vi "PhotonPoseEstimator_New.vi"(6 "BaseNTName":string="/photonvision", 8 "RobotToCamera":T1={"TRANSLATION3D"={"X"=0.0, "Y"=0.0, "Z"=0.0}, "ROTATION3D"={"Q_quaternion"={"R"=1.0, "V"=[0.0, 0.0, 0.0]}}, "XF"=FALSE} {"TRANSLATION3D"."Z" format="%14.3f"; "TRANSLATION3D"."Y" format="%14.3f"; "TRANSLATION3D"."X" format="%14.3f"}, 9 "Camera":string, 10 "Strategy":T5, 11 "AprilTagFieldLayout":T6={"AprilTagMap"={}, "FieldLength"=0.0, "FieldWidth"=0.0, "OriginPosition "=enum."kBlueAllianceWallRightSide,", "OriginPose3d"={"Translation3d"={"X"=0.0, "Y"=0.0, "Z"=0.0}, "Rotation3d"={"Q_quaternion"={"R"=1.0, "V"=[0.0, 0.0, 0.0]}}}} {"OriginPose3d"."Translation3d"."Z" format="%14.3f"; "OriginPose3d"."Translation3d"."Y" format="%14.3f"; "OriginPose3d"."Translation3d"."X" format="%14.3f"}) -> (3 "PhotonPoseEstimator":T10)   [LabVIEW 2019, in "PhotonVisionLib.lvlib"]
doc: "Create a new Photon Pose Estimator data cluster.\n\nThe PhotonPoseEstimator functions filters or combines readings from all the AprilTags visible at a given timestamp on the field to produce a single robot in field pose, using the strategy set below. Example usage can be found under the LabVIEW Find Examples..\n\nInputs:\n -- AprilTagFieldLayout -- cluster -- A WPILib LabVIEW Math cluster defining the absolute positions of April Tags on a FIRST field. with respect to the FIRST field \n -- Strategy -- Enum -- The strategy it should use to determine the best pose. Current strategies include:\n LOWEST_AMBIGUITY -- Choose the Pose with the lowest ambiguity\n CLOSEST_TO_CAMERA_HEIGHT -- Choose the Pose which is closest to the camera height.\n CLOSEST_TO_REFERENCE_POSE -- Choose the Pose which is closest to a set Reference position.\n CLOSEST_TO_LAST_POSE -- Choose the Pose which is closest to the last pose calculated\n AVERAGE_BEST_TARGETS -- Weight average of acceptable targets based on ambiguity..\n -- CameraName -- String -- Name of the photon camera.\n -- RobotToCamera -- Transform3d -- Transform from the center of the robot to the camera mount positions\n\nOutputs:\n -- PhotonPoseEstimator -- cluster -- created data cluster."
uses:
  PhotonVisionLib.lvlib
  Ref/PhotonPoseEstimator_REF.ctl
  TypeDef/PhotonPoseEstimatorType.ctl
  <vilib>/Rock Robotics/WPI/ThirdParty/JAS_Junk/TrajLib/TypeDef/POSE3D.ctl
  <vilib>/Rock Robotics/WPI/ThirdParty/JAS_Junk/TrajLib/TypeDef/TRANSLATION3D.ctl
  <vilib>/Rock Robotics/WPI/ThirdParty/JAS_Junk/TrajLib/TypeDef/ROTATION3D.ctl
  <vilib>/Rock Robotics/WPI/ThirdParty/JAS_Junk/TrajLib/TypeDef/QUATERNION.ctl
  <vilib>/Rock Robotics/WPI/ThirdParty/JAS_Junk/TrajLib/TypeDef/AprilTagFieldLayout.ctl
  <vilib>/Rock Robotics/WPI/ThirdParty/JAS_Junk/TrajLib/TypeDef/AprilTag.ctl
  <vilib>/Rock Robotics/WPI/ThirdParty/JAS_Junk/TrajLib/Enum/AprilTagFieldLayoutOrignPosition_ENUM.ctl
  Enum/PhotonPoseStrategy_ENUM.ctl
  <vilib>/Rock Robotics/WPI/ThirdParty/JAS_Junk/TrajLib/TypeDef/TRANSFORM3D.ctl
  TypeDef/PhotonTargetModel.ctl
  PhotonTargetModel_New_RectPlanar.vi
  <vilib>/Rock Robotics/WPI/ThirdParty/JAS_Junk/TrajLib/Conv_Inches_Meters.vi
  <vilib>/Rock Robotics/WPI/ThirdParty/JAS_Junk/TrajLib/VI/Translation3d_Create.vi
  PhotonTargetModel_New.vi
  <vilib>/Rock Robotics/WPI/ThirdParty/JAS_Junk/TrajLib/Trajectory_Library.lvlib
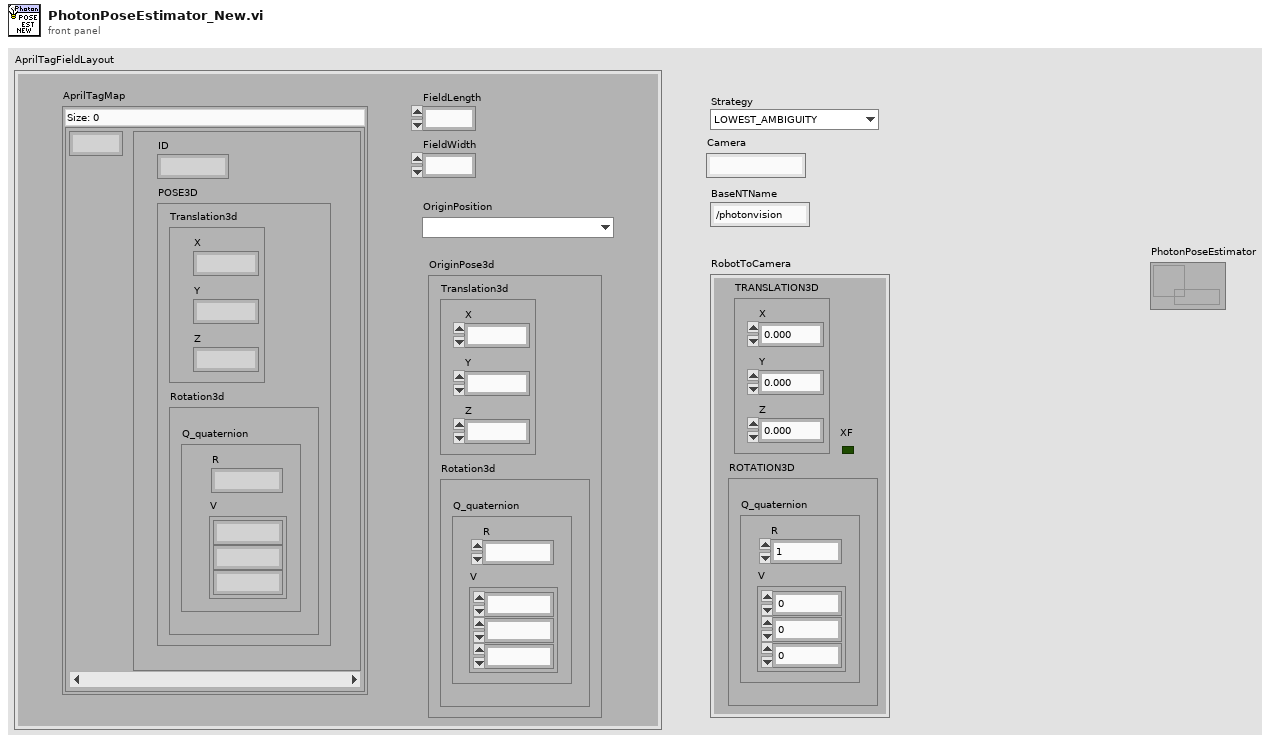
[diagram p1: front panel]
types:
  T1 = typedef "Trajectory_Library.lvlib/TRANSFORM3D.ctl" = cluster{"TRANSLATION3D":T2, "ROTATION3D":T3, "XF":bool}
  T2 = typedef "Trajectory_Library.lvlib/TRANSLATION3D.ctl" = cluster{"X":dbl, "Y":dbl, "Z":dbl}
  T3 = typedef "Trajectory_Library.lvlib/ROTATION3D.ctl" = cluster{"Q_quaternion":T4}
  T4 = typedef "Trajectory_Library.lvlib/QUATERNION.ctl" = cluster{"R":dbl, "V":dbl[]}
  T5 = typedef "PhotonVisionLib.lvlib/PhotonPoseStrategy_ENUM.ctl" = enum16{"LOWEST_AMBIGUITY", "CLOSEST_TO_CAMERA_HEIGHT", "CLOSEST_TO_REFERENCE_POSE", "CLOSEST_TO_LAST_POSE", "AVERAGE_BEST_TARGETS", "MULTI_TAG_PNP_ON_COPROCESSOR", "MULTI_TAG_PNP_ON_RIO"}
  T6 = typedef "Trajectory_Library.lvlib/AprilTagFieldLayout.ctl" = cluster{"AprilTagMap":map{i32, T7}, "FieldLength":dbl, "FieldWidth":dbl, "OriginPosition ":T9, "OriginPose3d":T8}
  T7 = typedef "Trajectory_Library.lvlib/AprilTag.ctl" = cluster{"ID":i32, "POSE3D":T8}
  T8 = typedef "Trajectory_Library.lvlib/POSE3D.ctl" = cluster{"Translation3d":T2, "Rotation3d":T3}
  T9 = typedef "Trajectory_Library.lvlib/AprilTagFieldLayoutOrignPosition_ENUM.ctl" = enum16{"kBlueAllianceWallRightSide,", "kRedAllianceWallRightSide,"}
  T10 = typedef "PhotonVisionLib.lvlib/PhotonPoseEstimator_REF.ctl" = refnum<data-value>
  T11 = typedef "PhotonVisionLib.lvlib/PhotonTargetModel.ctl" = cluster{"Vertices":T2[], "IsPlaner":bool, "IsSpherical":bool}
  T12 = typedef "PhotonVisionLib.lvlib/PhotonPoseEstimatorType.ctl" = cluster{"LastPose":T8, "ReferencePose":T8, "FieldTags":T6, "PrimaryStratety":T5, "Camera":string, "RobotToCamera":T1, "ReportedErrors":dbl[], "HighestAmbiguity":dbl, "MultiTagFallbackStrategy":T5, "PoseCacheTimeoutSec":dbl, "PhotonTargetModel":T11, "BaseNTName":string}
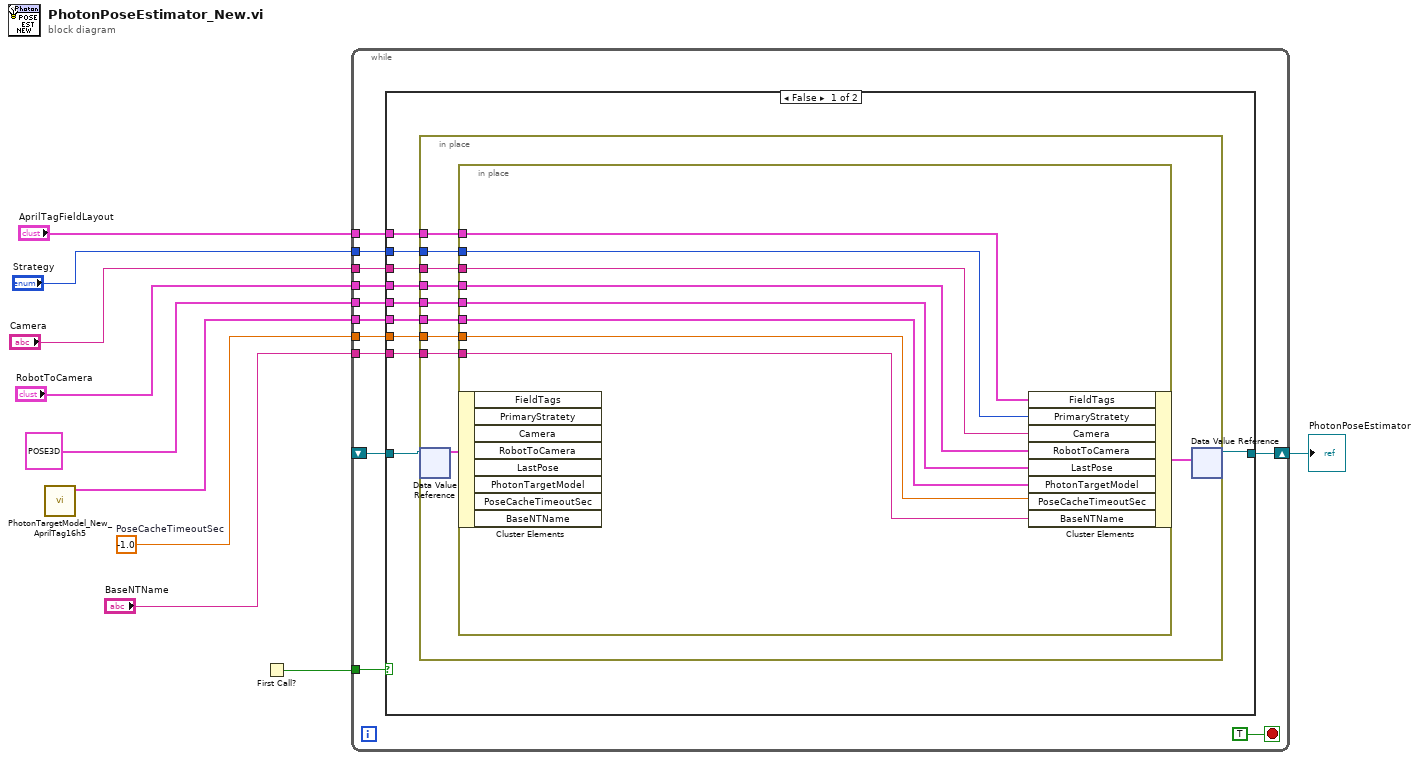
[diagram p0: block diagram]
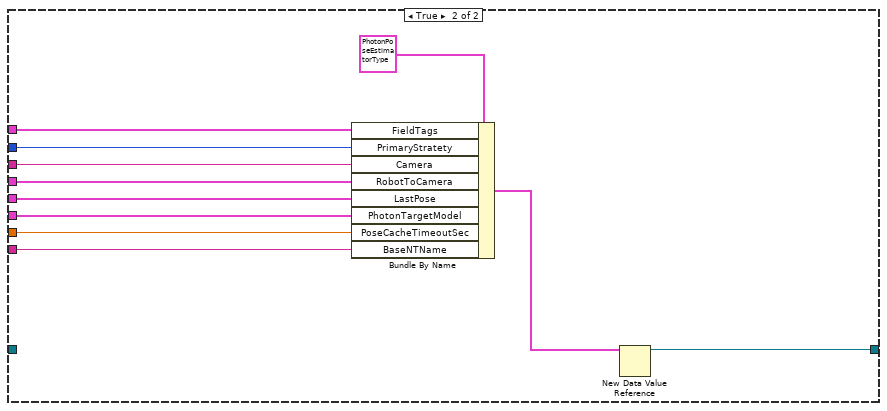
[diagram p2: hidden frame]
diagram:
  w4 = -1.0  # PoseCacheTimeoutSec
  n1 = call "PhotonTargetModel_New_AprilTag16h5.vi"() -> ("PhotonTargetModel"=w5:T11)  [unwired: 11 in]
  n2 = First Call?() -> (First Call?: T/F=w1:bool)
  n3 = while {
    tunnel: "AprilTagFieldLayout" -> [w22]
    tunnel: "Strategy" -> [w21]
    tunnel: "Camera" -> [w20]
    tunnel: "RobotToCamera" -> [w19]
    tunnel: T8 {"Translation3d"={"X"=0.0, "Y"=0.0, "Z"=0.0}, "Rotation3d"={"Q_quaternion"={"R"=1.0, "V"=[0.0, 0.0, 0.0]}}} ("LastPose") -> [w18]
    tunnel: w5 -> [w17]
    tunnel: w4 -> [w16]
    tunnel: "BaseNTName" -> [w15]
    tunnel: w1 -> [w13]
    shift-right: [w14] -> w2
    shift-left: _ -> [w11]
    stop <- TRUE stop-if-true
    n4 = case shown="False" w13 {
      tunnel: w22 -> [w30 w60]
      tunnel: w21 -> [w29 w59]
      tunnel: w20 -> [w28 w58]
      tunnel: w19 -> [w27 w57]
      tunnel: w18 -> [w26 w56]
      tunnel: w17 -> [w25 w55]
      tunnel: w16 -> [w24 w54]
      tunnel: w15 -> [w23 w53]
      tunnel: [w31 w51] -> w14
      tunnel: w11 -> [w32 _]
      frame False {
        n5 = in-place {
          in-place-border: w30 -> [w40]
          in-place-border: w29 -> [w39]
          in-place-border: w28 -> [w38]
          in-place-border: w27 -> [w37]
          in-place-border: w26 -> [w36]
          in-place-border: w25 -> [w35]
          in-place-border: w24 -> [w34]
          in-place-border: w23 -> [w33]
          n6 = in-place-dvr #1(w32) -> (w42:T12)  [unwired: 1 out]
          n7 = in-place {
            in-place-border: w40 -> [w50]
            in-place-border: w39 -> [w49]
            in-place-border: w38 -> [w48]
            in-place-border: w37 -> [w47]
            in-place-border: w36 -> [w46]
            in-place-border: w35 -> [w45]
            in-place-border: w34 -> [w44]
            in-place-border: w33 -> [w43]
            n8 = in-place-cluster #2(w42) -> ()  [unwired: 8 out]
            n9 = in-place-cluster #2("FieldTags"=w50, "PrimaryStratety"=w49, "Camera"=w48, "RobotToCamera"=w47, "LastPose"=w46, "PhotonTargetModel"=w45, "PoseCacheTimeoutSec"=w44, "BaseNTName"=w43) -> (w41:T12)
          }
          n10 = in-place-dvr #1(w41) -> (w31:refnum<data-value>)  [unwired: 1 out]
        }
      }
      frame True {
        n11 = Bundle By Name(cluster=T12 {"LastPose"={"Translation3d"={"X"=0.0, "Y"=0.0, "Z"=0.0}, "Rotation3d"={"Q_quaternion"={"R"=1.0, "V"=[0.0, 0.0, 0.0]}}}, "ReferencePose"={"Translation3d"={"X"=0.0, "Y"=0.0, "Z"=0.0}, "Rotation3d"={"Q_quaternion"={"R"=1.0, "V"=[0.0, 0.0, 0.0]}}}, "FieldTags"={"AprilTagMap"={}, "FieldLength"=0.0, "FieldWidth"=0.0, "OriginPosition "=enum."kBlueAllianceWallRightSide,", "OriginPose3d"={"Translation3d"={"X"=0.0, "Y"=0.0, "Z"=0.0}, "Rotation3d"={"Q_quaternion"={"R"=1.0, "V"=[0.0, 0.0, 0.0]}}}}, "PrimaryStratety"=enum."LOWEST_AMBIGUITY", "Camera"="", "RobotToCamera"={"TRANSLATION3D"={"X"=0.0, "Y"=0.0, "Z"=0.0}, "ROTATION3D"={"Q_quaternion"={"R"=1.0, "V"=[0.0, 0.0, 0.0]}}, "XF"=FALSE}, "ReportedErrors"=[], "HighestAmbiguity"=10.0, "MultiTagFallbackStrategy"=enum."LOWEST_AMBIGUITY", "PoseCacheTimeoutSec"=-1.0, "PhotonTargetModel"={"Vertices"=[], "IsPlaner"=FALSE, "IsSpherical"=FALSE}, "BaseNTName"="/photonvision"} ("PhotoPoseEstimator"), "FieldTags"=w60, "PrimaryStratety"=w59, "Camera"=w58, "RobotToCamera"=w57, "LastPose"=w56, "PhotonTargetModel"=w55, "PoseCacheTimeoutSec"=w54, "BaseNTName"=w53) -> (w52:T12)
        n12 = New Data Value Reference(data value=w52) -> (data value reference=w51:refnum<data-value>)  [unwired: 1 in, 1 out]
      }
    }
  }
  "PhotonPoseEstimator" <- w2
